vi "ConvertMaskToAlpha.vi"(11 "input cluster":T1) -> (3 "output cluster":T1)   [LabVIEW 2014, in "Raspberry Pi Compatible Compiler for LabVIEW.lvlib"]
uses:
  <vilib>/picture/picture.llb/imagedata.ctl
  Raspberry Pi Compatible Compiler for LabVIEW.lvlib
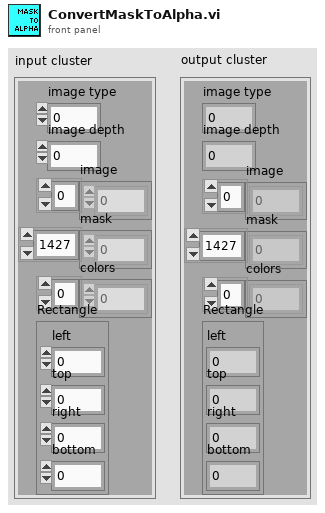
[diagram p1: front panel]
types:
  T1 = typedef "imagedata.ctl" = cluster{"image type":i32, "image depth":i32, "image":u8[], "mask":u8[], "colors":u32[], "Rectangle":cluster{"left":i16, "top":i16, "right":i16, "bottom":i16}}
  T2 = cluster{"left":i16, "top":i16, "right":i16, "bottom":i16}
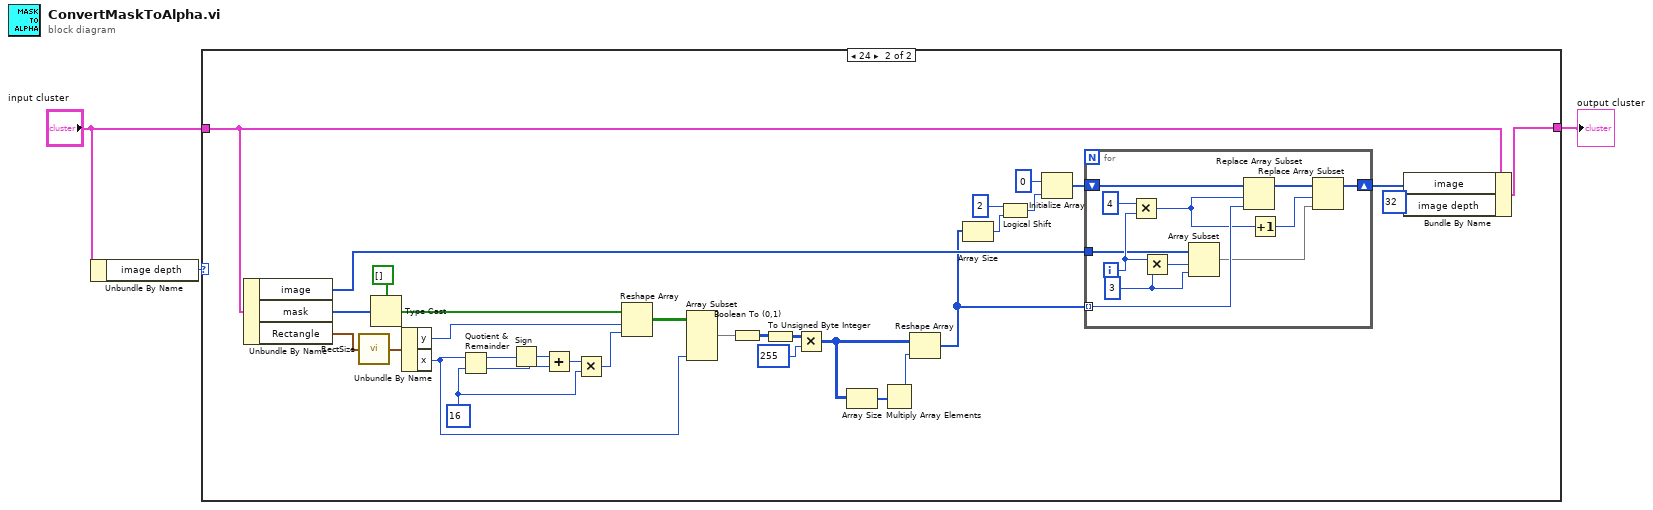
[diagram p0: block diagram]
diagram:
  n1 = Unbundle By Name("input cluster") -> ("image depth"=w1:i32)
  n2 = case shown="24" w1 {
    tunnel: "input cluster" -> [w4 w10]
    tunnel: [w4 w5] -> w3
    frame Default {
    }
    frame 24 {
      w28 = i16 16 ("y")
      n3 = Unbundle By Name(w10) -> ("image"=w22:u8[], "mask"=w36:u8[], "Rectangle"=w34:T2)
      n4 = call <vilib>:"RectSize.vi"("rect"=w34) -> ("point"=w33:cluster{"x":i16, "y":i16})
      n5 = Type Cast(type=bool[] [], x=w36) -> (*(type *) &x=w27:bool[])
      n6 = Unbundle By Name(w33) -> ("y"=w21:i16, "x"=w18:i16)
      n7 = Quotient & Remainder(x=w18, y=w28) -> (x-y*floor(x/y)=w32:i16, floor(x/y)=w30:i16)
      n8 = Sign(1:w32) -> (0:w31:i16)
      n9 = Add(x=w31, y=w30) -> (x+y=w29:i16)
      n10 = Multiply(x=w29, y=w28) -> (x*y=w26:i16)
      n11 = Reshape Array(w27, w21, w26) -> (w20:bool[][])
      n12 = Array Subset(array=w20, length (col)=w18) -> (w19:bool[][])  [unwired: 3 in]
      n13 = Boolean To (0,1)(Boolean=w19) -> (0, 1=w25:i16[][])
      n14 = To Unsigned Byte Integer(number=w25) -> (unsigned 8bit integer=w24:u8[][])
      n15 = Multiply(x=w24, y=u8 255) -> (x*y=w17:u8[][])
      n16 = Array Size(array=w17) -> (size(s)=w16:i32[])
      n17 = Multiply Array Elements(1:w16) -> (0:w12:i32)
      n18 = Reshape Array(w17, w12) -> (w6:u8[])
      n19 = Array Size(array=w6) -> (size(s)=w7:i32)
      n20 = Logical Shift(y=i16 2, x=w7) -> (x << y=w13:i32)
      n21 = Initialize Array(u8 0, w13) -> (w15:u8[])
      n22 = for {
        tunnel: w22 -> [w44]
        tunnel: w6 -> [w42] mode=indexing
        shift-right: [w40] -> w9
        shift-left: w15 -> [w48]
        i -> [w47]
        w43 = 3 ("y")
        n23 = Multiply(x=4 ("y"), y=w47) -> (x*y=w38:i32)
        n24 = Multiply(x=w47, y=w43) -> (x*y=w45:i32)
        n25 = Array Subset(array=w44, index=w45, length=w43) -> (w39:u8[])
        n26 = Replace Array Subset(array=w48, new element=w42, index=w38) -> (w41:u8[])
        n27 = Increment(x=w38) -> (x+1=w37:i32)
        n28 = Replace Array Subset(array=w41, new element=w39, index=w37) -> (w40:u8[])
      }
      n29 = Bundle By Name(cluster=w10, "image"=w9, "image depth"=32) -> (w5:T1)
    }
  }
  "output cluster" <- w3
